vi "Mux4Way16.vi"(0 "a":bool[](array[boolean])=[FALSE, FALSE, FALSE, FALSE, FALSE, FALSE, FALSE, FALSE, FALSE, FALSE, FALSE, FALSE, FALSE, FALSE, FALSE, FALSE], 2 "b":bool[](array[boolean])=[FALSE, FALSE, FALSE, FALSE, FALSE, FALSE, FALSE, FALSE, FALSE, FALSE, FALSE, FALSE, FALSE, FALSE, FALSE, FALSE], 3 "c":bool[](array[boolean])=[FALSE, FALSE, FALSE, FALSE, FALSE, FALSE, FALSE, FALSE, FALSE, FALSE, FALSE, FALSE, FALSE, FALSE, FALSE, FALSE], 4 "sel":bool[](array[boolean])=[FALSE, FALSE], 5 "d":bool[](array[boolean])=[FALSE, FALSE, FALSE, FALSE, FALSE, FALSE, FALSE, FALSE, FALSE, FALSE, FALSE, FALSE, FALSE, FALSE, FALSE, FALSE]) -> (7 "out":bool[](array[boolean]))   [LabVIEW 2014]
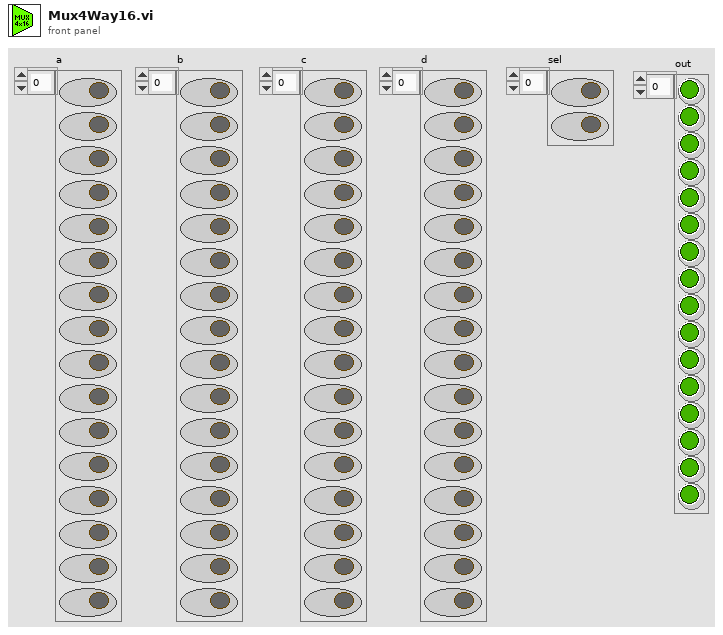
[diagram p1: front panel]
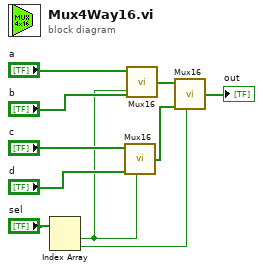
[diagram p0: block diagram]
diagram:
  n1 = Index Array(array="sel") -> (element #1=w3:bool, element #2=w2:bool)  [unwired: 2 in]
  n2 = call "Mux16.vi"("a"="c", "sel"=w3, "b"="d") -> ("out"=w5:bool[])  [unwired: 5 in]
  n3 = call "Mux16.vi"("a"="a", "sel"=w3, "b"="b") -> ("out"=w6:bool[])  [unwired: 5 in]
  n4 = call "Mux16.vi"("a"=w6, "sel"=w2, "b"=w5) -> ("out"=→"out":bool[])  [unwired: 5 in]
